vi "RTEH Sort and Convert Ranges.vi"(8 "error in (no error)":errorcluster, 10 "Error Display Options":T3[](array[typedef])) -> (0 "error out":errorcluster, 1 "Detect Any Warnings":bool, 2 "Error Processing Options":T1[](array[typedef]), 4 "Valid Default":bool, 6 "Default Action":T1)   [LabVIEW 2017]
uses:
  <userlib>/_SEH/Controls/RTEH/RTEH Error Display Options.ctl
  <userlib>/_SEH/Controls/RTEH/RTEH Shared Error Options.ctl
  <userlib>/_SEH/Controls/RTEH/RTEH Error Options.ctl
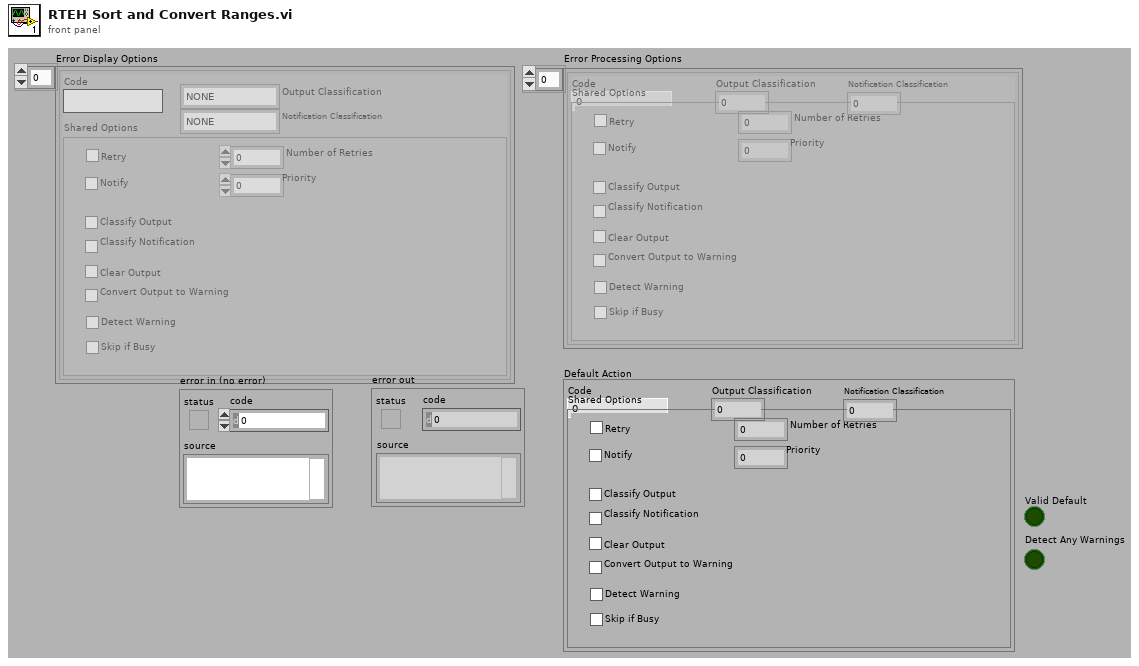
[diagram p1: front panel]
types:
  T1 = typedef "RTEH Error Options.ctl" = cluster{"Code":i32, "Shared Options":T2, "Output Classification":u32, "Notification Classification":u32}
  T2 = typedef "RTEH Shared Error Options.ctl" = cluster{"Number of Retries":i32, "Retry":bool, "Classify Output":bool, "Classify Notification":bool, "Convert Output to Warning":bool, "Clear Output":bool, "Notify":bool, "Priority":i32, "Detect Warning":bool, "Skip if Busy":bool}
  T3 = typedef "RTEH Error Display Options.ctl" = cluster{"Code":string, "Shared Options":T2, "Output Classification":string, "Notification Classification":string}
  T4 = typedef "SEH Code Types.ctl" = enum16{"Code", "Range", "Category", "Invalid", "Default Action"}
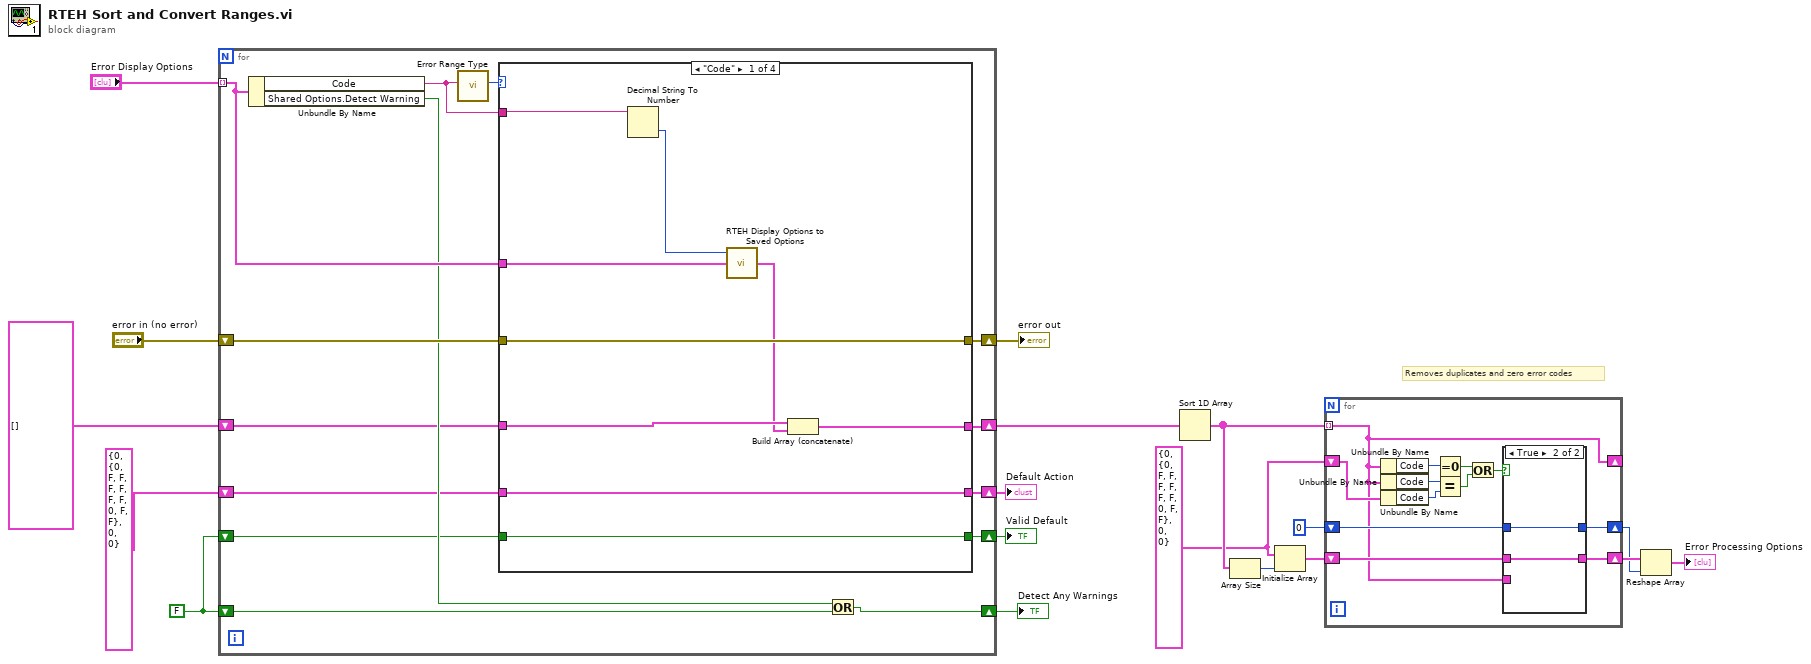
[diagram p0: block diagram]
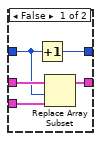
[diagram p2: hidden frame]
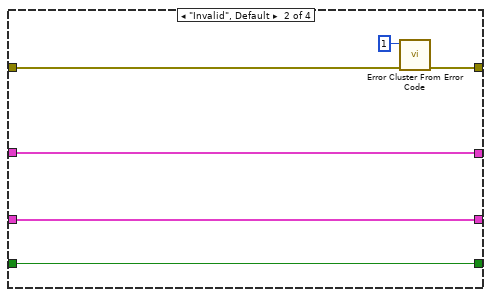
[diagram p3: hidden frame]
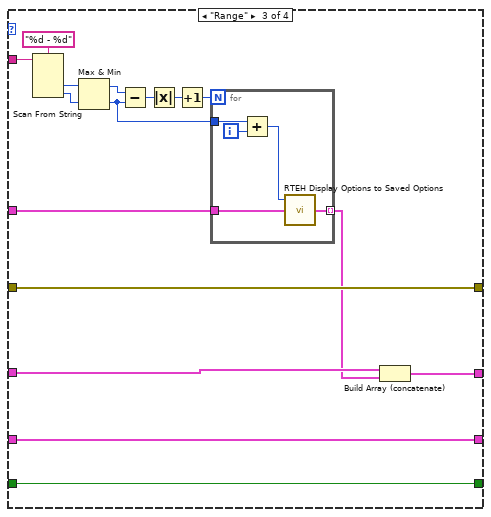
[diagram p4: hidden frame]
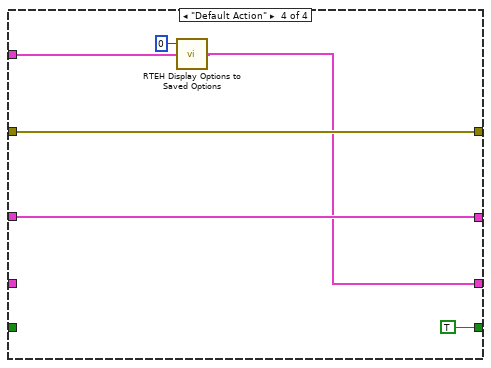
[diagram p5: hidden frame]
diagram:
  w3 = FALSE
  w15 = T1 {"Code"=0, "Shared Options"={"Number of Retries"=0, "Retry"=FALSE, "Classify Output"=FALSE, "Classify Notification"=FALSE, "Convert Output to Warning"=FALSE, "Clear Output"=FALSE, "Notify"=FALSE, "Priority"=0, "Detect Warning"=FALSE, "Skip if Busy"=FALSE}, "Output Classification"=0, "Notification Classification"=0} ("Error Options")
  # "Removes duplicates and zero error codes"
  n1 = for {
    tunnel: "Error Display Options" -> [w30] mode=indexing
    shift-right: [w28] -> w8
    shift-left: "error in (no error)" -> [w29]
    shift-right: [w25] -> w7
    shift-left: w3 -> [w26]
    shift-right: [w23] -> w5
    shift-left: T1[] [] -> [w24]
    shift-right: [w20] -> w2
    shift-left: T1 {"Code"=0, "Shared Options"={"Number of Retries"=0, "Retry"=FALSE, "Classify Output"=FALSE, "Classify Notification"=FALSE, "Convert Output to Warning"=FALSE, "Clear Output"=FALSE, "Notify"=FALSE, "Priority"=0, "Detect Warning"=FALSE, "Skip if Busy"=FALSE}, "Output Classification"=0, "Notification Classification"=0} ("Shared Options") -> [w21]
    shift-right: [w19] -> w1
    shift-left: w3 -> [w22]
    n2 = Unbundle By Name(w30) -> ("Code"=w31:string, "Shared Options.Detect Warning"=w27:bool)
    n3 = call <userlib>:"Error Range Type.vi"("Codes"=w31) -> ("Type"=w32:T4)  [unwired: 10 out]
    n4 = case shown="\"Code\"" w32 {
      tunnel: w31 -> [w41 _ w63 _]
      tunnel: w30 -> [w38 _ w58 w74]
      tunnel: w29 -> [w40 w47 w53 w72]
      tunnel: [w40 w46 w53 w72] -> w28
      tunnel: w24 -> [w37 w44 w52 w71]
      tunnel: [w35 w44 w50 w71] -> w23
      tunnel: w22 -> [w33 w42 w49 _]
      tunnel: w21 -> [w34 w43 w48 _]
      tunnel: [w34 w43 w48 w69] -> w20
      tunnel: [w33 w42 w49 TRUE] -> w19
      frame "Code" {
        n5 = Decimal String To Number(string=w41) -> (number=w39:i32)  [unwired: 3 out]
        n6 = call <userlib>:"RTEH Display Options to Saved Options.vi"("Display Error Options"=w38, "Code"=w39) -> ("Saved Error Options"=w36:T1)  [unwired: 1 in]
        n7 = Build Array (concatenate)(w37, w36) -> (w35:T1[])
      }
      frame "Invalid", Default {
        n8 = call <vilib>:"Error Cluster From Error Code.vi"("error in (no error)"=w47, "error code (0)"=1) -> ("error out"=w46:errorcluster)  [unwired: 1 in, 6 out]
      }
      frame "Range" {
        n9 = Scan From String(format string="%d - %d", input string=w63) -> (output 1=w61:i32, output 2=w60:i32)  [unwired: 2 in, 5 out]
        n10 = Max & Min(x=w61, y=w60) -> (max(x,y)=w57:i32, min(x,y)=w56:i32)
        n11 = Subtract(x=w57, y=w56) -> (x-y=w59:i32)
        n12 = Absolute Value(x=w59) -> (abs(x)=w55:i32)
        n13 = Increment(x=w55) -> (x+1=w54:i32)
        n14 = for {
          N: w54 -> [_]
          tunnel: w58 -> [w64]
          tunnel: w56 -> [w68]
          tunnel: [w65] -> w51 mode=indexing
          i -> [w67]
          n15 = Add(x=w68, y=w67) -> (x+y=w66:i32)
          n16 = call <userlib>:"RTEH Display Options to Saved Options.vi"("Display Error Options"=w64, "Code"=w66) -> ("Saved Error Options"=w65:T1)  [unwired: 1 in]
        }
        n17 = Build Array (concatenate)(w52, w51) -> (w50:T1[])
      }
      frame "Default Action" {
        n18 = call <userlib>:"RTEH Display Options to Saved Options.vi"("Display Error Options"=w74, "Code"=0) -> ("Saved Error Options"=w69:T1)  [unwired: 1 in]
      }
    }
    n19 = Or(x=w27, y=w26) -> (x .or. y?=w25:bool)
  }
  "error out" <- w8
  "Detect Any Warnings" <- w7
  "Default Action" <- w2
  "Valid Default" <- w1
  n20 = Sort 1D Array(array=w5) -> (sorted array=w16:T1[])
  n21 = Array Size(array=w16) -> (size(s)=w14:i32)
  n22 = Initialize Array(w15, w14) -> (w13:T1[])
  n23 = for {
    tunnel: w16 -> [w75] mode=indexing
    shift-right: [w75] -> _
    shift-left: w15 -> [w84]
    shift-right: [w78] -> w11
    shift-left: 0 -> [w79]
    shift-right: [w76] -> w12
    shift-left: w13 -> [w77]
    n24 = Unbundle By Name(w75) -> ("Code"=w83:i32)
    n25 = Unbundle By Name(w75) -> ("Code"=w86:i32)
    n26 = Unbundle By Name(w84) -> ("Code"=w85:i32)
    n27 = Equal To 0?(x=w83) -> (x = 0?=w82:bool)
    n28 = Equal?(x=w86, y=w85) -> (x = y?=w81:bool)
    n29 = Or(x=w82, y=w81) -> (x .or. y?=w80:bool)
    n30 = case shown="True" w80 {
      tunnel: w79 -> [w88 w92]
      tunnel: [w91 w92] -> w78
      tunnel: w77 -> [w90 w93]
      tunnel: [w89 w93] -> w76
      tunnel: w75 -> [w87 _]
      frame False {
        n31 = Increment(x=w88) -> (x+1=w91:i32)
        n32 = Replace Array Subset(array=w90, new element=w87, index=w88) -> (w89:T1[])
      }
      frame True {
      }
    }
  }
  n33 = Reshape Array(w12, w11) -> (→"Error Processing Options":T1[])
